vi "Set Voltage.vi"(8 "error in (no error)":errorcluster, 9 "V Range (12: 1000)":u16(ring)=12 items=["AUTO", "1.5", "3", "6", "10", "15", "30", "60", "100", "150", "300", "600", "1000"], 10 "Element (0: All)":u16(ring) items=["All", "Element 1", "Element 2", "Element 3", "Element 4", "Element 5", "Element 6"], 11 "Universal Power Meter in":refnum<class "Universal Power Meter.lvclass">) -> (0 "error out":errorcluster, 2 "Power Meter Visa":refnum<visa-resource-name>, 3 "Universal Power Meter out":refnum<class "Universal Power Meter.lvclass">)   [LabVIEW 2012, in "Universal Power Meter.lvlib" / "Universal Power Meter.lvclass"]
uses:
  Universal Power Meter.lvclass
  Universal Power Meter.lvclass/Universal Power Meter.ctl
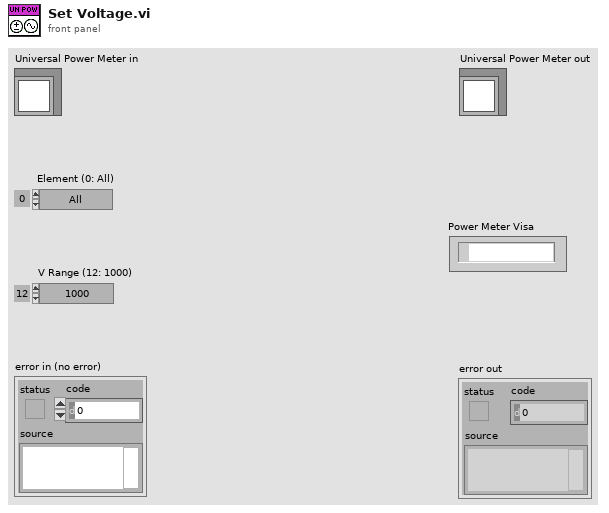
[diagram p1: front panel]
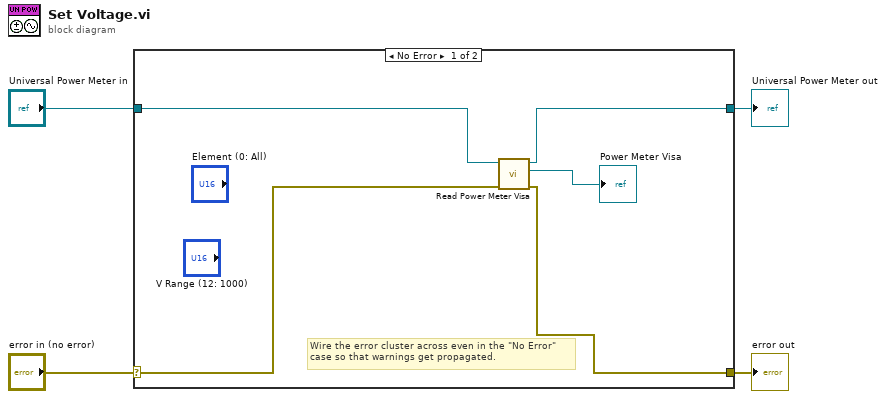
[diagram p0: block diagram]
diagram:
  n1 = case shown="No Error" "error in (no error)" {
    selector: "error in (no error)" -> [w6 w11]
    tunnel: [w5 w11] -> w3
    tunnel: [w8 w10] -> w1
    tunnel: "Universal Power Meter in" -> [w9 w10]
    frame No Error {
      # "Wire the error cluster across even in the \"No Error\"\ncase so that warnings get propagated."
      n2 = call "Read Power Meter Visa.vi"("error in (no error)"=w6, "Universal Power Meter in"=w9) -> ("error out"=w5:errorcluster, "Power Meter Visa"=→"Power Meter Visa":refnum<visa-resource-name>, "Universal Power Meter out"=w8:refnum<class "Universal Power Meter.lvclass">)  [unwired: 7 in]
    }
    frame Error {
    }
  }
  "error out" <- w3
  "Universal Power Meter out" <- w1
